vi "Playback.vi"(11 "Playback":bool) -> (3 "Outputs":T1={"Slider 1"=0.0, "Slider 2"=-0.007874015748031496})   [LabVIEW 2012]
uses:
  Downloads/Team 1736 Autoflex v1.1 %28Fixed%29 (1)/Joystick Event.ctl
panel:
  out "Info Path":path=path "C:/Users/FRC/Desktop/Autoflex/000.txt"
  in  "Inputs":T1={"Slider 1"=0.0, "Slider 2"=-0.007874015748031496}
  out "Joystick Event":cluster{"Timestamp":u32, "Input":T1}={"Timestamp"=657367, "Input"={"Slider 1"=0.0, "Slider 2"=-0.007874015748031496}}
  out "Joystick Event Array":cluster{"Timestamp":u32, "Input":T1}[](array[cluster])=[{"Timestamp"=234633, "Input"={"Slider 1"=-0.047244094488188976, "Slider 2"=0.0}}, {"Timestamp"=234778, "Input"={"Slider 1"=-0.08661417322834646, "Slider 2"=-0.06299212598425197}}, {"Timestamp"=234848, "Input"={"Slider 1"=-0.08661417322834646, "Slider 2"=-0.14173228346456693}}, {"Timestamp"=234900, "Input"={"Slider 1"=-0.10236220472440945, "Slider 2"=-0.18110236220472442}}, {"Timestamp"=234954, "Input"={"Slider 1"=-0.12598425196850394, "Slider 2"=-0.28346456692913385}}, {"Timestamp"=235026, "Input"={"Slider 1"=-0.12598425196850394, "Slider 2"=-0.3228346456692913}}, {"Timestamp"=235372, "Input"={"Slider 1"=-0.12598425196850394, "Slider 2"=-0.3464566929133858}}, {"Timestamp"=235433, "Input"={"Slider 1"=0.07874015748031496, "Slider 2"=-0.4015748031496063}}, {"Timestamp"=235492, "Input"={"Slider 1"=-0.16535433070866143, "Slider 2"=-0.44881889763779526}}, {"Timestamp"=235557, "Input"={"Slider 1"=-0.18110236220472442, "Slider 2"=-0.4881889763779528}}, {"Timestamp"=235623, "Input"={"Slider 1"=-0.18110236220472442, "Slider 2"=-0.5039370078740157}}, {"Timestamp"=236417, "Input"={"Slider 1"=-0.18110236220472442, "Slider 2"=-0.30708661417322836}}, {"Timestamp"=236495, "Input"={"Slider 1"=0.0, "Slider 2"=-0.023622047244094488}}, {"Timestamp"=236541, "Input"={"Slider 1"=0.0, "Slider 2"=-0.007874015748031496}}, {"Timestamp"=236695, "Input"={"Slider 1"=0.0, "Slider 2"=0.0}}, {"Timestamp"=236902, "Input"={"Slider 1"=0.0, "Slider 2"=0.031496062992125984}}, {"Timestamp"=236955, "Input"={"Slider 1"=0.03937007874015748, "Slider 2"=0.09448818897637795}}, {"Timestamp"=237014, "Input"={"Slider 1"=0.11811023622047244, "Slider 2"=0.1732283464566929}}, {"Timestamp"=237078, "Input"={"Slider 1"=0.023622047244094488, "Slider 2"=0.2755905511811024}}, {"Timestamp"=237136, "Input"={"Slider 1"=0.0, "Slider 2"=0.3543307086614173}}, {"Timestamp"=237217, "Input"={"Slider 1"=0.0, "Slider 2"=0.4566929133858268}}, {"Timestamp"=237272, "Input"={"Slider 1"=0.0, "Slider 2"=0.5196850393700787}}, {"Timestamp"=237332, "Input"={"Slider 1"=0.0, "Slider 2"=0.5433070866141733}}, {"Timestamp"=237398, "Input"={"Slider 1"=0.0, "Slider 2"=0.5590551181102362}}, {"Timestamp"=237460, "Input"={"Slider 1"=0.0, "Slider 2"=0.5826771653543307}}, {"Timestamp"=237774, "Input"={"Slider 1"=0.0, "Slider 2"=0.5039370078740157}}, {"Timestamp"=237798, "Input"={"Slider 1"=0.0, "Slider 2"=0.4566929133858268}}, {"Timestamp"=237854, "Input"={"Slider 1"=0.0, "Slider 2"=0.31496062992125984}}, {"Timestamp"=237914, "Input"={"Slider 1"=0.0, "Slider 2"=0.05511811023622047}}, {"Timestamp"=237973, "Input"={"Slider 1"=0.0, "Slider 2"=0.0}}, {"Timestamp"=238179, "Input"={"Slider 1"=-0.023622047244094488, "Slider 2"=0.0}}, {"Timestamp"=238417, "Input"={"Slider 1"=-0.047244094488188976, "Slider 2"=-0.007874015748031496}}, {"Timestamp"=238454, "Input"={"Slider 1"=-0.06299212598425197, "Slider 2"=-0.007874015748031496}}, {"Timestamp"=238577, "Input"={"Slider 1"=-0.06299212598425197, "Slider 2"=-0.047244094488188976}}, {"Timestamp"=238615, "Input"={"Slider 1"=-0.08661417322834646, "Slider 2"=-0.08661417322834646}}, {"Timestamp"=238761, "Input"={"Slider 1"=-0.10236220472440945, "Slider 2"=-0.3464566929133858}}, {"Timestamp"=238815, "Input"={"Slider 1"=-0.16535433070866143, "Slider 2"=-0.3858267716535433}}, {"Timestamp"=238937, "Input"={"Slider 1"=0.0, "Slider 2"=-0.4015748031496063}}, {"Timestamp"=238999, "Input"={"Slider 1"=-0.16535433070866143, "Slider 2"=-0.44881889763779526}}, {"Timestamp"=239062, "Input"={"Slider 1"=-0.16535433070866143, "Slider 2"=-0.4645669291338583}}, {"Timestamp"=239362, "Input"={"Slider 1"=-0.08661417322834646, "Slider 2"=-0.4645669291338583}}, {"Timestamp"=239439, "Input"={"Slider 1"=-0.08661417322834646, "Slider 2"=-0.3858267716535433}}, {"Timestamp"=239476, "Input"={"Slider 1"=-0.08661417322834646, "Slider 2"=-0.2677165354330709}}, {"Timestamp"=239513, "Input"={"Slider 1"=-0.06299212598425197, "Slider 2"=-0.16535433070866143}}, {"Timestamp"=239553, "Input"={"Slider 1"=-0.047244094488188976, "Slider 2"=-0.14173228346456693}}, {"Timestamp"=239592, "Input"={"Slider 1"=0.0, "Slider 2"=-0.08661417322834646}}, {"Timestamp"=239644, "Input"={"Slider 1"=0.0, "Slider 2"=-0.007874015748031496}}, {"Timestamp"=239722, "Input"={"Slider 1"=0.03937007874015748, "Slider 2"=-0.007874015748031496}}, {"Timestamp"=239757, "Input"={"Slider 1"=0.0, "Slider 2"=-0.007874015748031496}}, {"Timestamp"=489779, "Input"={"Slider 1"=-0.023622047244094488, "Slider 2"=-0.007874015748031496}}, {"Timestamp"=489877, "Input"={"Slider 1"=-0.023622047244094488, "Slider 2"=-0.03937007874015748}}, {"Timestamp"=489894, "Input"={"Slider 1"=-0.023622047244094488, "Slider 2"=-0.07086614173228346}}, {"Timestamp"=489919, "Input"={"Slider 1"=-0.03937007874015748, "Slider 2"=-0.11811023622047244}}, {"Timestamp"=489939, "Input"={"Slider 1"=-0.05511811023622047, "Slider 2"=-0.14960629921259844}}, {"Timestamp"=489980, "Input"={"Slider 1"=-0.07874015748031496, "Slider 2"=-0.25196850393700787}}, {"Timestamp"=490002, "Input"={"Slider 1"=-0.03937007874015748, "Slider 2"=-0.2992125984251969}}, {"Timestamp"=490038, "Input"={"Slider 1"=-0.03937007874015748, "Slider 2"=-0.3858267716535433}}, {"Timestamp"=490060, "Input"={"Slider 1"=-0.09448818897637795, "Slider 2"=-0.4015748031496063}}, {"Timestamp"=490099, "Input"={"Slider 1"=-0.14960629921259844, "Slider 2"=-0.4330708661417323}}, {"Timestamp"=490217, "Input"={"Slider 1"=-0.16535433070866143, "Slider 2"=-0.44881889763779526}}, {"Timestamp"=490237, "Input"={"Slider 1"=-0.16535433070866143, "Slider 2"=-0.4645669291338583}}, {"Timestamp"=490279, "Input"={"Slider 1"=-0.16535433070866143, "Slider 2"=-0.48031496062992124}}, {"Timestamp"=490317, "Input"={"Slider 1"=-0.16535433070866143, "Slider 2"=-0.49606299212598426}}, {"Timestamp"=490336, "Input"={"Slider 1"=-0.16535433070866143, "Slider 2"=-0.5118110236220472}}, {"Timestamp"=490357, "Input"={"Slider 1"=-0.16535433070866143, "Slider 2"=-0.5354330708661418}}, {"Timestamp"=490380, "Input"={"Slider 1"=-0.16535433070866143, "Slider 2"=-0.5511811023622047}}, {"Timestamp"=490419, "Input"={"Slider 1"=-0.1889763779527559, "Slider 2"=-0.5511811023622047}}, {"Timestamp"=490475, "Input"={"Slider 1"=-0.1889763779527559, "Slider 2"=-0.5669291338582677}}, {"Timestamp"=490498, "Input"={"Slider 1"=-0.2047244094488189, "Slider 2"=-0.5669291338582677}}, {"Timestamp"=490557, "Input"={"Slider 1"=-0.2204724409448819, "Slider 2"=-0.5669291338582677}}, {"Timestamp"=490739, "Input"={"Slider 1"=-0.2204724409448819, "Slider 2"=-0.4645669291338583}}, {"Timestamp"=490764, "Input"={"Slider 1"=-0.2204724409448819, "Slider 2"=-0.41732283464566927}}, {"Timestamp"=490785, "Input"={"Slider 1"=-0.2204724409448819, "Slider 2"=-0.3464566929133858}}, {"Timestamp"=490816, "Input"={"Slider 1"=-0.16535433070866143, "Slider 2"=-0.11811023622047244}}, {"Timestamp"=490839, "Input"={"Slider 1"=0.0, "Slider 2"=-0.03937007874015748}}, {"Timestamp"=490882, "Input"={"Slider 1"=0.0, "Slider 2"=-0.007874015748031496}}, {"Timestamp"=490934, "Input"={"Slider 1"=0.0, "Slider 2"=0.0}}, {"Timestamp"=490958, "Input"={"Slider 1"=0.15748031496062992, "Slider 2"=0.0}}, {"Timestamp"=490980, "Input"={"Slider 1"=0.0, "Slider 2"=0.0}}, {"Timestamp"=491056, "Input"={"Slider 1"=0.0, "Slider 2"=0.007874015748031496}}, {"Timestamp"=491122, "Input"={"Slider 1"=0.0, "Slider 2"=0.03937007874015748}}, {"Timestamp"=491143, "Input"={"Slider 1"=0.0, "Slider 2"=0.05511811023622047}}, {"Timestamp"=491175, "Input"={"Slider 1"=0.0, "Slider 2"=0.11811023622047244}}, {"Timestamp"=491196, "Input"={"Slider 1"=0.0, "Slider 2"=0.14960629921259844}}, {"Timestamp"=491217, "Input"={"Slider 1"=0.0, "Slider 2"=0.18110236220472442}}, {"Timestamp"=491237, "Input"={"Slider 1"=0.0, "Slider 2"=0.2125984251968504}}, {"Timestamp"=491262, "Input"={"Slider 1"=-0.05511811023622047, "Slider 2"=0.25196850393700787}}, {"Timestamp"=491297, "Input"={"Slider 1"=-0.07874015748031496, "Slider 2"=0.3937007874015748}}, {"Timestamp"=491332, "Input"={"Slider 1"=-0.09448818897637795, "Slider 2"=0.4251968503937008}}, {"Timestamp"=491355, "Input"={"Slider 1"=-0.09448818897637795, "Slider 2"=0.5196850393700787}}, {"Timestamp"=491416, "Input"={"Slider 1"=-0.03937007874015748, "Slider 2"=0.5196850393700787}}, {"Timestamp"=491496, "Input"={"Slider 1"=-0.09448818897637795, "Slider 2"=0.5196850393700787}}, {"Timestamp"=491598, "Input"={"Slider 1"=-0.11023622047244094, "Slider 2"=0.5196850393700787}}, {"Timestamp"=491657, "Input"={"Slider 1"=-0.14960629921259844, "Slider 2"=0.5196850393700787}}, {"Timestamp"=491717, "Input"={"Slider 1"=-0.16535433070866143, "Slider 2"=0.5196850393700787}}, {"Timestamp"=491858, "Input"={"Slider 1"=-0.11023622047244094, "Slider 2"=0.5196850393700787}}, {"Timestamp"=491894, "Input"={"Slider 1"=-0.09448818897637795, "Slider 2"=0.5196850393700787}}, {"Timestamp"=491943, "Input"={"Slider 1"=-0.07874015748031496, "Slider 2"=0.5196850393700787}}, {"Timestamp"=491977, "Input"={"Slider 1"=-0.05511811023622047, "Slider 2"=0.4094488188976378}}, {"Timestamp"=491996, "Input"={"Slider 1"=-0.05511811023622047, "Slider 2"=0.3937007874015748}}, {"Timestamp"=492036, "Input"={"Slider 1"=-0.05511811023622047, "Slider 2"=0.3464566929133858}}, {"Timestamp"=492058, "Input"={"Slider 1"=-0.05511811023622047, "Slider 2"=0.2992125984251969}}, {"Timestamp"=492082, "Input"={"Slider 1"=-0.03937007874015748, "Slider 2"=0.2677165354330709}}, {"Timestamp"=492116, "Input"={"Slider 1"=-0.03937007874015748, "Slider 2"=0.16535433070866143}}, {"Timestamp"=492178, "Input"={"Slider 1"=-0.09448818897637795, "Slider 2"=0.16535433070866143}}, {"Timestamp"=492481, "Input"={"Slider 1"=-0.09448818897637795, "Slider 2"=0.14960629921259844}}, {"Timestamp"=492495, "Input"={"Slider 1"=-0.09448818897637795, "Slider 2"=0.13385826771653545}}, {"Timestamp"=492519, "Input"={"Slider 1"=-0.09448818897637795, "Slider 2"=0.11811023622047244}}, {"Timestamp"=492540, "Input"={"Slider 1"=-0.09448818897637795, "Slider 2"=0.07086614173228346}}, {"Timestamp"=492574, "Input"={"Slider 1"=-0.03937007874015748, "Slider 2"=0.03937007874015748}}, {"Timestamp"=492623, "Input"={"Slider 1"=-0.03937007874015748, "Slider 2"=0.007874015748031496}}, {"Timestamp"=492666, "Input"={"Slider 1"=-0.023622047244094488, "Slider 2"=0.0}}, {"Timestamp"=492715, "Input"={"Slider 1"=0.0, "Slider 2"=0.0}}, {"Timestamp"=492736, "Input"={"Slider 1"=0.0, "Slider 2"=-0.007874015748031496}}, {"Timestamp"=492805, "Input"={"Slider 1"=-0.09448818897637795, "Slider 2"=-0.023622047244094488}}, {"Timestamp"=492836, "Input"={"Slider 1"=-0.09448818897637795, "Slider 2"=-0.10236220472440945}}, {"Timestamp"=492864, "Input"={"Slider 1"=-0.16535433070866143, "Slider 2"=-0.13385826771653545}}, {"Timestamp"=492898, "Input"={"Slider 1"=-0.2047244094488189, "Slider 2"=-0.2047244094488189}}, {"Timestamp"=492921, "Input"={"Slider 1"=-0.2204724409448819, "Slider 2"=-0.25196850393700787}}, {"Timestamp"=492937, "Input"={"Slider 1"=-0.2204724409448819, "Slider 2"=-0.2992125984251969}}, {"Timestamp"=492960, "Input"={"Slider 1"=-0.2204724409448819, "Slider 2"=-0.31496062992125984}}, {"Timestamp"=492996, "Input"={"Slider 1"=-0.2755905511811024, "Slider 2"=-0.33070866141732286}}, {"Timestamp"=493016, "Input"={"Slider 1"=-0.2992125984251969, "Slider 2"=-0.33070866141732286}}, {"Timestamp"=493079, "Input"={"Slider 1"=-0.2440944881889764, "Slider 2"=-0.33070866141732286}}, {"Timestamp"=493103, "Input"={"Slider 1"=-0.2047244094488189, "Slider 2"=-0.33070866141732286}}, {"Timestamp"=493118, "Input"={"Slider 1"=-0.2047244094488189, "Slider 2"=-0.2677165354330709}}, {"Timestamp"=493141, "Input"={"Slider 1"=-0.2047244094488189, "Slider 2"=-0.2204724409448819}}, {"Timestamp"=493175, "Input"={"Slider 1"=-0.1889763779527559, "Slider 2"=-0.14960629921259844}}, {"Timestamp"=493202, "Input"={"Slider 1"=-0.16535433070866143, "Slider 2"=-0.11811023622047244}}, {"Timestamp"=493238, "Input"={"Slider 1"=-0.09448818897637795, "Slider 2"=-0.03937007874015748}}, {"Timestamp"=493266, "Input"={"Slider 1"=-0.03937007874015748, "Slider 2"=-0.023622047244094488}}, {"Timestamp"=493300, "Input"={"Slider 1"=0.0, "Slider 2"=-0.007874015748031496}}, {"Timestamp"=493415, "Input"={"Slider 1"=-0.05511811023622047, "Slider 2"=-0.07086614173228346}}, {"Timestamp"=493442, "Input"={"Slider 1"=-0.05511811023622047, "Slider 2"=-0.11811023622047244}}, {"Timestamp"=493479, "Input"={"Slider 1"=-0.09448818897637795, "Slider 2"=-0.2677165354330709}}, {"Timestamp"=493498, "Input"={"Slider 1"=-0.09448818897637795, "Slider 2"=-0.4015748031496063}}, {"Timestamp"=493517, "Input"={"Slider 1"=-0.14960629921259844, "Slider 2"=-0.44881889763779526}}, {"Timestamp"=493543, "Input"={"Slider 1"=-0.1889763779527559, "Slider 2"=-0.48031496062992124}}, {"Timestamp"=493567, "Input"={"Slider 1"=-0.2204724409448819, "Slider 2"=-0.48031496062992124}}, {"Timestamp"=493698, "Input"={"Slider 1"=-0.16535433070866143, "Slider 2"=-0.48031496062992124}}, {"Timestamp"=493727, "Input"={"Slider 1"=-0.16535433070866143, "Slider 2"=-0.41732283464566927}}, {"Timestamp"=493754, "Input"={"Slider 1"=-0.16535433070866143, "Slider 2"=-0.33070866141732286}}, {"Timestamp"=493776, "Input"={"Slider 1"=-0.14960629921259844, "Slider 2"=-0.2047244094488189}}, {"Timestamp"=493795, "Input"={"Slider 1"=-0.13385826771653545, "Slider 2"=-0.11811023622047244}}, {"Timestamp"=493817, "Input"={"Slider 1"=-0.05511811023622047, "Slider 2"=-0.023622047244094488}}, {"Timestamp"=493836, "Input"={"Slider 1"=0.0, "Slider 2"=-0.007874015748031496}}, {"Timestamp"=494162, "Input"={"Slider 1"=0.0, "Slider 2"=0.0}}, {"Timestamp"=494184, "Input"={"Slider 1"=0.0, "Slider 2"=0.007874015748031496}}, {"Timestamp"=494224, "Input"={"Slider 1"=0.0, "Slider 2"=0.023622047244094488}}, {"Timestamp"=494238, "Input"={"Slider 1"=0.0, "Slider 2"=0.03937007874015748}}, {"Timestamp"=494277, "Input"={"Slider 1"=0.0, "Slider 2"=0.07086614173228346}}, {"Timestamp"=494299, "Input"={"Slider 1"=0.0, "Slider 2"=0.11811023622047244}}, {"Timestamp"=494337, "Input"={"Slider 1"=0.0, "Slider 2"=0.14960629921259844}}, {"Timestamp"=494361, "Input"={"Slider 1"=0.0, "Slider 2"=0.1968503937007874}}, {"Timestamp"=494400, "Input"={"Slider 1"=0.0, "Slider 2"=0.2992125984251969}}, {"Timestamp"=494416, "Input"={"Slider 1"=0.0, "Slider 2"=0.36220472440944884}}, {"Timestamp"=494439, "Input"={"Slider 1"=0.0, "Slider 2"=0.3937007874015748}}, {"Timestamp"=494458, "Input"={"Slider 1"=0.0, "Slider 2"=0.4251968503937008}}, {"Timestamp"=494476, "Input"={"Slider 1"=0.0, "Slider 2"=0.47244094488188976}}, {"Timestamp"=494502, "Input"={"Slider 1"=0.0, "Slider 2"=0.5039370078740157}}, {"Timestamp"=494543, "Input"={"Slider 1"=0.0, "Slider 2"=0.5196850393700787}}, {"Timestamp"=494578, "Input"={"Slider 1"=0.0, "Slider 2"=0.5354330708661418}}, {"Timestamp"=494613, "Input"={"Slider 1"=0.0, "Slider 2"=0.5511811023622047}}, {"Timestamp"=494647, "Input"={"Slider 1"=0.0, "Slider 2"=0.5669291338582677}}, {"Timestamp"=494737, "Input"={"Slider 1"=0.0, "Slider 2"=0.5039370078740157}}, {"Timestamp"=494776, "Input"={"Slider 1"=0.0, "Slider 2"=0.4409448818897638}}, {"Timestamp"=494798, "Input"={"Slider 1"=-0.03937007874015748, "Slider 2"=0.4409448818897638}}, {"Timestamp"=494835, "Input"={"Slider 1"=-0.07874015748031496, "Slider 2"=0.4094488188976378}}, {"Timestamp"=494856, "Input"={"Slider 1"=-0.09448818897637795, "Slider 2"=0.3937007874015748}}, {"Timestamp"=494896, "Input"={"Slider 1"=-0.09448818897637795, "Slider 2"=0.31496062992125984}}, {"Timestamp"=494918, "Input"={"Slider 1"=-0.03937007874015748, "Slider 2"=0.23622047244094488}}, {"Timestamp"=494937, "Input"={"Slider 1"=0.0, "Slider 2"=0.05511811023622047}}, {"Timestamp"=494961, "Input"={"Slider 1"=0.0, "Slider 2"=0.0}}, {"Timestamp"=494976, "Input"={"Slider 1"=0.0, "Slider 2"=-0.007874015748031496}}, {"Timestamp"=495102, "Input"={"Slider 1"=-0.05511811023622047, "Slider 2"=-0.007874015748031496}}, {"Timestamp"=495230, "Input"={"Slider 1"=-0.07874015748031496, "Slider 2"=-0.023622047244094488}}, {"Timestamp"=495256, "Input"={"Slider 1"=-0.07874015748031496, "Slider 2"=-0.10236220472440945}}, {"Timestamp"=495284, "Input"={"Slider 1"=-0.09448818897637795, "Slider 2"=-0.13385826771653545}}, {"Timestamp"=495334, "Input"={"Slider 1"=-0.13385826771653545, "Slider 2"=-0.25196850393700787}}, {"Timestamp"=495358, "Input"={"Slider 1"=-0.1889763779527559, "Slider 2"=-0.41732283464566927}}, {"Timestamp"=495400, "Input"={"Slider 1"=-0.2440944881889764, "Slider 2"=-0.5118110236220472}}, {"Timestamp"=495436, "Input"={"Slider 1"=-0.2992125984251969, "Slider 2"=-0.5669291338582677}}, {"Timestamp"=495459, "Input"={"Slider 1"=-0.2992125984251969, "Slider 2"=-0.6141732283464567}}, {"Timestamp"=495497, "Input"={"Slider 1"=-0.31496062992125984, "Slider 2"=-0.6614173228346457}}, {"Timestamp"=495519, "Input"={"Slider 1"=-0.31496062992125984, "Slider 2"=-0.6771653543307087}}, {"Timestamp"=495672, "Input"={"Slider 1"=-0.31496062992125984, "Slider 2"=-0.6141732283464567}}, {"Timestamp"=495694, "Input"={"Slider 1"=-0.31496062992125984, "Slider 2"=-0.5354330708661418}}, {"Timestamp"=495722, "Input"={"Slider 1"=-0.31496062992125984, "Slider 2"=-0.48031496062992124}}, {"Timestamp"=495759, "Input"={"Slider 1"=-0.2047244094488189, "Slider 2"=-0.25196850393700787}}, {"Timestamp"=495776, "Input"={"Slider 1"=-0.14960629921259844, "Slider 2"=-0.10236220472440945}}, {"Timestamp"=495817, "Input"={"Slider 1"=0.0, "Slider 2"=-0.007874015748031496}}, {"Timestamp"=495903, "Input"={"Slider 1"=0.0, "Slider 2"=0.0}}, {"Timestamp"=495998, "Input"={"Slider 1"=0.0, "Slider 2"=0.023622047244094488}}, {"Timestamp"=496022, "Input"={"Slider 1"=0.0, "Slider 2"=0.05511811023622047}}, {"Timestamp"=496076, "Input"={"Slider 1"=0.0, "Slider 2"=0.13385826771653545}}, {"Timestamp"=496100, "Input"={"Slider 1"=0.0, "Slider 2"=0.1968503937007874}}, {"Timestamp"=496141, "Input"={"Slider 1"=0.0, "Slider 2"=0.31496062992125984}}, {"Timestamp"=496181, "Input"={"Slider 1"=0.0, "Slider 2"=0.4094488188976378}}, {"Timestamp"=496227, "Input"={"Slider 1"=0.0, "Slider 2"=0.5196850393700787}}, {"Timestamp"=496556, "Input"={"Slider 1"=-0.05511811023622047, "Slider 2"=0.5196850393700787}}, {"Timestamp"=496598, "Input"={"Slider 1"=-0.05511811023622047, "Slider 2"=0.4409448818897638}}, {"Timestamp"=496615, "Input"={"Slider 1"=-0.05511811023622047, "Slider 2"=0.4094488188976378}}, {"Timestamp"=496635, "Input"={"Slider 1"=-0.05511811023622047, "Slider 2"=0.3779527559055118}}, {"Timestamp"=496657, "Input"={"Slider 1"=-0.05511811023622047, "Slider 2"=0.2992125984251969}}, {"Timestamp"=496696, "Input"={"Slider 1"=-0.05511811023622047, "Slider 2"=0.023622047244094488}}, {"Timestamp"=496716, "Input"={"Slider 1"=-0.05511811023622047, "Slider 2"=-0.007874015748031496}}, {"Timestamp"=653789, "Input"={"Slider 1"=0.0, "Slider 2"=-0.007874015748031496}}]
  out "Array size":i32=207
  out "Last Played Index":i32
  out "Retrieve Index":i32
  out "Start Time":u32
  out "File Path":path=path "C:/Users/FRC/Desktop/Autoflex/000.autoflex"
  out "Next Joystick Event":cluster{"Timestamp":u32, "Input":T1}
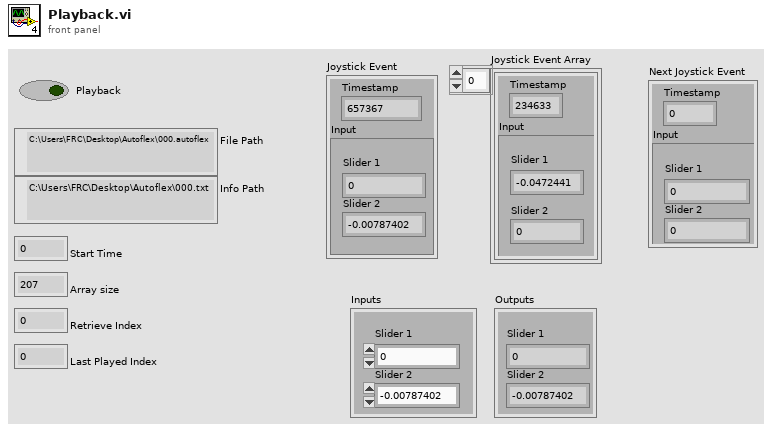
[diagram p1: front panel]
types:
  T1 = typedef "Joystick Event.ctl" = cluster{"Slider 1":dbl, "Slider 2":dbl}
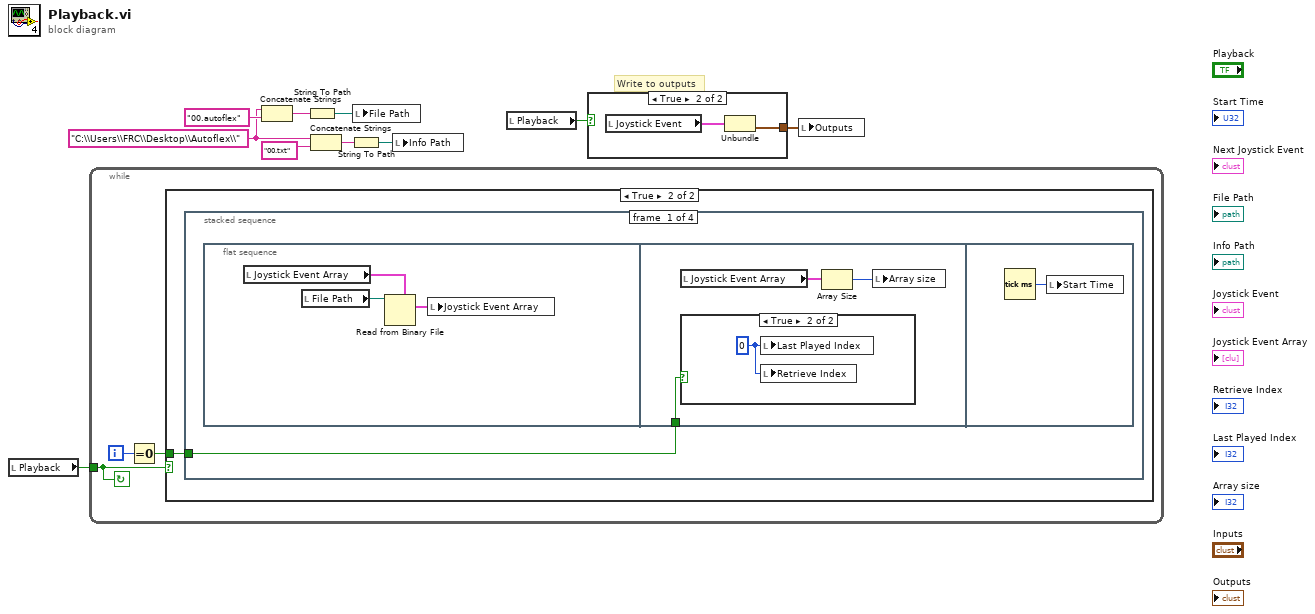
[diagram p0: block diagram]
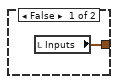
[diagram p2: hidden frame]
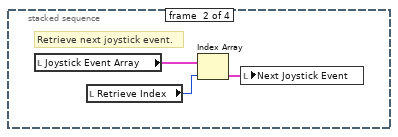
[diagram p5: hidden frame]
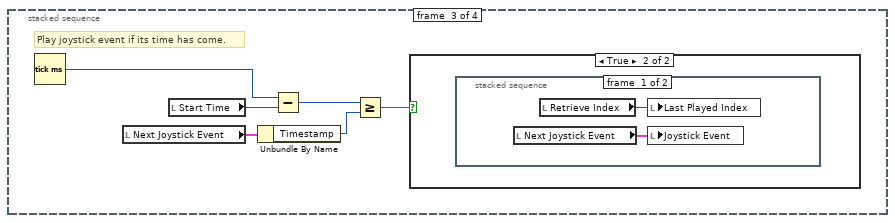
[diagram p6: hidden frame]
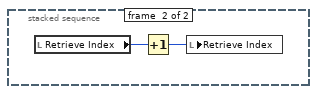
[diagram p8: hidden frame]
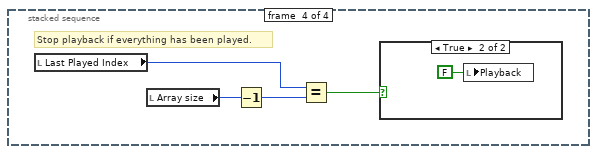
[diagram p9: hidden frame]
diagram:
  w1 = "C:\\Users\\FRC\\Desktop\\Autoflex\\" ("string")
  # "Write to outputs"
  n1 = local read "Playback"() -> (w10:bool)
  n2 = while {
    tunnel: w10 -> [w13]
    i -> [w12]
    stop <- w13 continue-if-true
    n3 = Equal To 0?(x=w12) -> (x = 0?=w11:bool)
    n4 = case shown="True" w13 {
      tunnel: w11 -> [_ w14]
      frame False {
      }
      frame True {
        n5 = stacked-sequence {
          tunnel: w14 -> [w15 _ _ _]
          frame #0 {
            n6 = flat-sequence {
              tunnel: w15 -> [w19]
              frame #0 {
                n7 = local read "Joystick Event Array"() -> (w17:cluster{"Timestamp":u32, "Input":T1}[])
                n8 = local read "File Path"() -> (w16:path)
                n9 = Read from Binary File(5:w17, 11:w16) -> (2:w18:cluster{"Timestamp":u32, "Input":T1}[])  [unwired: 1 in, 6 out]
                n10 = local write "Joystick Event Array"(w18) -> ()
              }
              frame #1 {
                n11 = local read "Joystick Event Array"() -> (w20:cluster{"Timestamp":u32, "Input":T1}[])
                n12 = case shown="True" w19 {
                  frame False {
                  }
                  frame True {
                    w22 = 0 ("index")
                    n13 = local write "Last Played Index"(w22) -> ()
                    n14 = local write "Retrieve Index"(w22) -> ()
                  }
                }
                n15 = Array Size(array=w20) -> (size(s)=w21:i32)
                n16 = local write "Array size"(w21) -> ()
              }
              frame #2 {
                n17 = Tick Count (ms)() -> (millisecond timer value=w23:u32)
                n18 = local write "Start Time"(w23) -> ()
              }
            }
          }
          frame #1 {
            # "Retrieve next joystick event."
            n19 = local read "Joystick Event Array"() -> (w25:cluster{"Timestamp":u32, "Input":T1}[])
            n20 = local read "Retrieve Index"() -> (w26:i32)
            n21 = Index Array(array=w25, index=w26) -> (element=w24:cluster{"Timestamp":u32, "Input":T1})
            n22 = local write "Next Joystick Event"(w24) -> ()
          }
          frame #2 {
            # "Play joystick event if its time has come."
            n23 = Tick Count (ms)() -> (millisecond timer value=w28:u32)
            n24 = local read "Next Joystick Event"() -> (w30:cluster{"Timestamp":u32, "Input":T1})
            n25 = local read "Start Time"() -> (w27:u32)
            n26 = Unbundle By Name(w30) -> ("Timestamp"=w29:u32)
            n27 = Subtract(x=w28, y=w27) -> (x-y=w31:u32)
            n28 = Greater Or Equal?(x=w31, y=w29) -> (x >= y?=w32:bool)
            n29 = case shown="True" w32 {
              frame False {
              }
              frame True {
                n30 = stacked-sequence {
                  frame #0 {
                    n31 = local read "Next Joystick Event"() -> (w33:cluster{"Timestamp":u32, "Input":T1})
                    n32 = local read "Retrieve Index"() -> (w34:i32)
                    n33 = local write "Last Played Index"(w34) -> ()
                    n34 = local write "Joystick Event"(w33) -> ()
                  }
                  frame #1 {
                    n35 = local read "Retrieve Index"() -> (w36:i32)
                    n36 = Increment(x=w36) -> (x+1=w35:i32)
                    n37 = local write "Retrieve Index"(w35) -> ()
                  }
                }
              }
            }
          }
          frame #3 {
            # "Stop playback if everything has been played."
            n38 = local read "Last Played Index"() -> (w37:i32)
            n39 = local read "Array size"() -> (w38:i32)
            n40 = Decrement(x=w38) -> (x-1=w40:i32)
            n41 = Equal?(x=w37, y=w40) -> (x = y?=w39:bool)
            n42 = case shown="True" w39 {
              frame False {
              }
              frame True {
                n43 = local write "Playback"(FALSE ("Playback Button")) -> ()
              }
            }
          }
        }
      }
    }
  }
  n44 = Concatenate Strings(w1, "00.autoflex" ("string")) -> (w4:string)
  n45 = String To Path(string=w4) -> (path=w6:path)
  n46 = Concatenate Strings(w1, "00.txt" ("string")) -> (w3:string)
  n47 = String To Path(string=w3) -> (path=w5:path)
  n48 = local write "File Path"(w6) -> ()
  n49 = local write "Info Path"(w5) -> ()
  n50 = local read "Playback"() -> (w9:bool)
  n51 = case shown="True" w9 {
    tunnel: [w42 w43] -> w8
    frame False {
      n52 = local read "Inputs"() -> (w42:T1)
    }
    frame True {
      n53 = local read "Joystick Event"() -> (w44:cluster{"Timestamp":u32, "Input":T1})
      n54 = Unbundle(w44) -> ("Input"=w43:T1)  [unwired: 1 out]
    }
  }
  n55 = local write "Outputs"(w8) -> ()
